vi "Ejercicio_2_3.vi"() -> ()   [LabVIEW 2020]
panel:
  out "Thermometer":dbl(slide) scale=0.0..100.0
  out "Numeric 2":i32
  out "Numeric":i32
  out "Tank":dbl(slide) scale=0.0..10.0
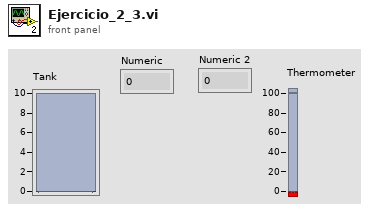
[diagram p1: front panel]
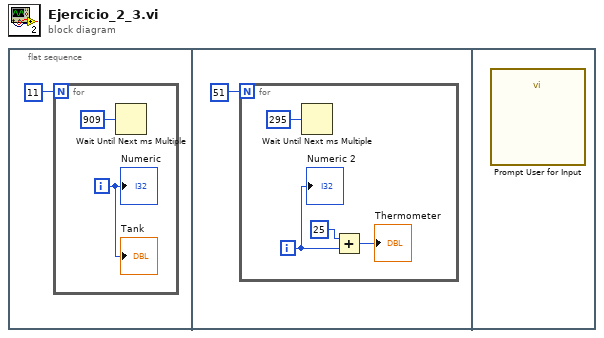
[diagram p0: block diagram]
diagram:
  n1 = flat-sequence {
    frame #0 {
      n2 = for {
        N: 11 -> [_]
        i -> [w2]
        n3 = Wait Until Next ms Multiple(millisecond multiple=909) -> ()  [unwired: 1 out]
        "Tank" <- w2
        "Numeric" <- w2
      }
    }
    frame #1 {
      n4 = for {
        N: 51 -> [_]
        i -> [w6]
        n5 = Wait Until Next ms Multiple(millisecond multiple=295) -> ()  [unwired: 1 out]
        n6 = Add(x=25, y=w6) -> (x+y=→"Thermometer":i32)
        "Numeric 2" <- w6
      }
    }
    frame #2 {
      n7 = call "Prompt User for Input"() -> ()  [unwired: 18 in, 2 out]
    }
  }
